vi "Preserving Class Values.vi"(10 "Format":T1, 11 "File in":refnum<class "File.lvclass">) -> (3 "File out":refnum<class "File.lvclass">)   [LabVIEW 2020, in "Manejador archivo.lvlib"]
uses:
  Manejador archivo.lvlib
  Class Definitions/File/File.lvclass
  File Formats--enum.ctl
  Class Definitions/TDMS/TDMS.lvclass
  C:/GitClones/DQMH-LabVIEW-GYM/10 Mayo/04 DQMH USER/Libraries/Manejador archivo/Class Definitions/File/File.lvclass
  Class Definitions/File/File.lvclass/File.ctl
  Class Definitions/CSV/CSV.lvclass
  Class Definitions/File/Read Column Headers.vi
  Class Definitions/File/Read Delimiter.vi
  Class Definitions/File/Read File Path.vi
  Class Definitions/File/Read Save Timestamp.vi
  Class Definitions/File/Write Column Headers.vi
  Class Definitions/File/Write Delimiter.vi
  Class Definitions/File/Write File Path.vi
  Class Definitions/File/Write Save Timestamp.vi
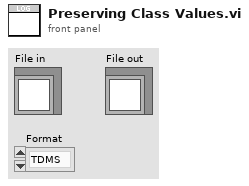
[diagram p1: front panel]
types:
  T1 = typedef "Manejador archivo.lvlib/File Formats--enum.ctl" = enum16{"TDMS", "CSV"}
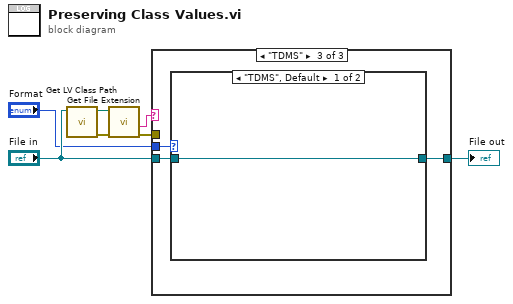
[diagram p0: block diagram]
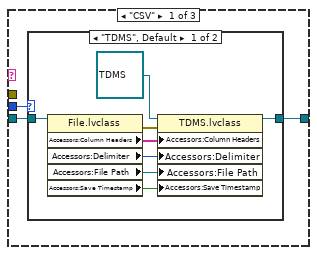
[diagram p2: hidden frame]
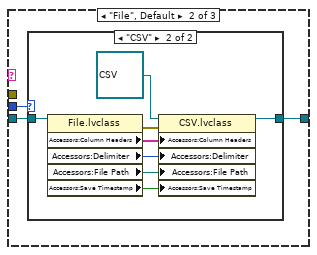
[diagram p4: hidden frame]
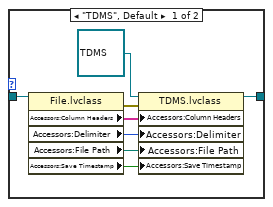
[diagram p5: hidden frame]
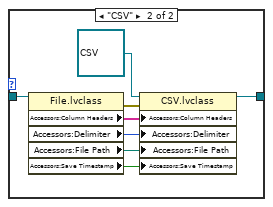
[diagram p6: hidden frame]
diagram:
  n1 = call <vilib>:"Get LV Class Path.vi"("object"="File in") -> ("error out"=w4:errorcluster, "class path"=w3:path)  [unwired: 9 in]
  n2 = call <vilib>:"Get File Extension.vi"("error in (no error)"=w4, "file"=w3) -> ("error out"=w2:errorcluster, "filename without extension"=w1:string)  [unwired: 5 in, 3 out]
  n3 = case shown="\"TDMS\"" w1 {
    tunnel: w2 -> [_ _ _]
    tunnel: "File in" -> [w9 w21 w40]
    tunnel: [w8 w20 w39] -> w7
    tunnel: "Format" -> [w10 w22 w41]
    frame "CSV" {
      n4 = case shown="\"TDMS\", Default" w10 {
        tunnel: w9 -> [w16 w19]
        tunnel: [w17 w19] -> w8
        frame "TDMS", Default {
          n5 = property class="File.lvclass"(reference=w16) -> (error out=w11:errorcluster, "Accessors:Column Headers"=w12:string[], "Accessors:Delimiter"=w13:enum16{"Tab", "Coma"}, "Accessors:File Path"=w14:path, "Accessors:Save Timestamp"=w15:bool)  [unwired: 1 in, 1 out]
          n6 = property class="TDMS.lvclass"(reference=refnum<class "TDMS.lvclass"> refnum ("Manejador archivo.lvlib:TDMS.lvclass"), error in=w11, "Accessors:Column Headers"=w12, "Accessors:Delimiter"=w13, "Accessors:File Path"=w14, "Accessors:Save Timestamp"=w15) -> (reference out=w17:refnum<class "TDMS.lvclass">)  [unwired: 1 out]
        }
        frame "CSV" {
        }
      }
    }
    frame "File", Default {
      n7 = case shown="\"CSV\"" w22 {
        tunnel: w21 -> [w28 w37]
        tunnel: [w29 w38] -> w20
        frame "TDMS", Default {
          n8 = property class="File.lvclass"(reference=w28) -> (error out=w23:errorcluster, "Accessors:Column Headers"=w24:string[], "Accessors:Delimiter"=w25:enum16{"Tab", "Coma"}, "Accessors:File Path"=w26:path, "Accessors:Save Timestamp"=w27:bool)  [unwired: 1 in, 1 out]
          n9 = property class="TDMS.lvclass"(reference=refnum<class "TDMS.lvclass"> refnum ("Manejador archivo.lvlib:TDMS.lvclass"), error in=w23, "Accessors:Column Headers"=w24, "Accessors:Delimiter"=w25, "Accessors:File Path"=w26, "Accessors:Save Timestamp"=w27) -> (reference out=w29:refnum<class "TDMS.lvclass">)  [unwired: 1 out]
        }
        frame "CSV" {
          n10 = property class="File.lvclass"(reference=w37) -> (error out=w32:errorcluster, "Accessors:Column Headers"=w33:string[], "Accessors:Delimiter"=w34:enum16{"Tab", "Coma"}, "Accessors:File Path"=w35:path, "Accessors:Save Timestamp"=w36:bool)  [unwired: 1 in, 1 out]
          n11 = property class="CSV.lvclass"(reference=refnum<class "CSV.lvclass"> refnum ("Manejador archivo.lvlib:CSV.lvclass"), error in=w32, "Accessors:Column Headers"=w33, "Accessors:Delimiter"=w34, "Accessors:File Path"=w35, "Accessors:Save Timestamp"=w36) -> (reference out=w38:refnum<class "CSV.lvclass">)  [unwired: 1 out]
        }
      }
    }
    frame "TDMS" {
      n12 = case shown="\"TDMS\", Default" w41 {
        tunnel: w40 -> [w42 w49]
        tunnel: [w42 w50] -> w39
        frame "TDMS", Default {
        }
        frame "CSV" {
          n13 = property class="File.lvclass"(reference=w49) -> (error out=w44:errorcluster, "Accessors:Column Headers"=w45:string[], "Accessors:Delimiter"=w46:enum16{"Tab", "Coma"}, "Accessors:File Path"=w47:path, "Accessors:Save Timestamp"=w48:bool)  [unwired: 1 in, 1 out]
          n14 = property class="CSV.lvclass"(reference=refnum<class "CSV.lvclass"> refnum ("Manejador archivo.lvlib:CSV.lvclass"), error in=w44, "Accessors:Column Headers"=w45, "Accessors:Delimiter"=w46, "Accessors:File Path"=w47, "Accessors:Save Timestamp"=w48) -> (reference out=w50:refnum<class "CSV.lvclass">)  [unwired: 1 out]
        }
      }
    }
  }
  "File out" <- w7
